vi "PV HLT5xx Valve Test.vi"(6 "Auto/Manual in":bool[](array[boolean]), 7 "Adress of unit":u16=1 min=1 max=999 step=1, 8 "error in (no error)":errorcluster, 9 "On/Off in":bool[](array[boolean]), 10 "Parameter\nread only<->describe":bool, 11 "VISA session":refnum<visa-resource-name>) -> (0 "error out":errorcluster, 1 "On/Off out":bool[](array[boolean]), 2 "response (data)":string, 3 "dup VISA session":refnum<visa-resource-name>, 4 "Auto/Manual out":bool[](array[boolean]))   [LabVIEW 2016, in "Pfeiffer Vacuum.lvlib"]
doc: "This VI allows you to set or check the Valve \"Valve test (Para 609)\" on the SmartTest (HLT5xx)."
uses:
  Pfeiffer Vacuum.lvlib
panel:
  # "Valve test"
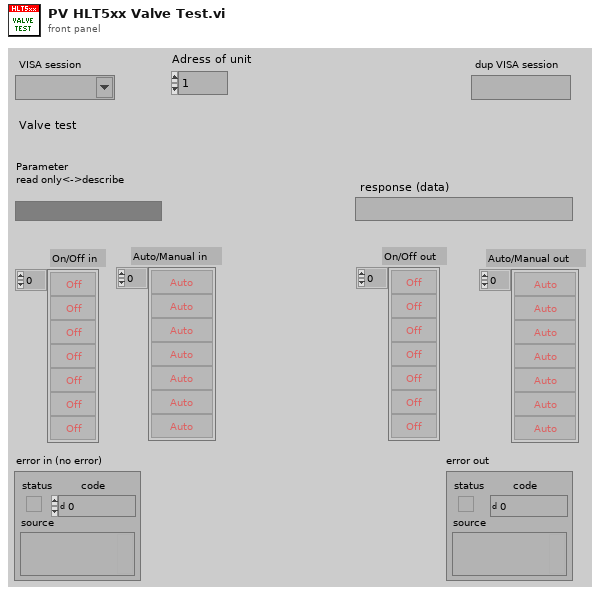
[diagram p1: front panel]
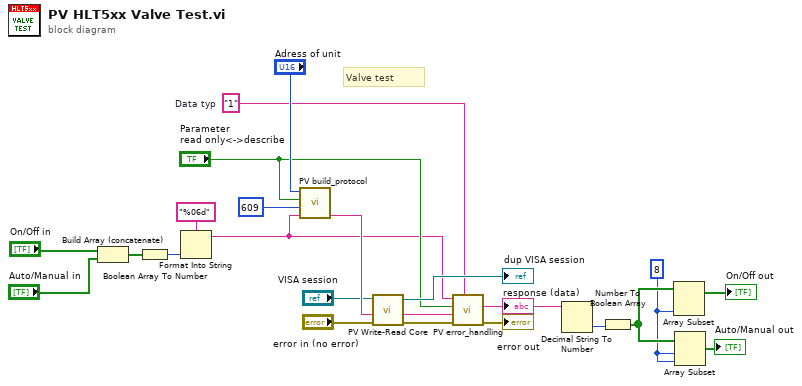
[diagram p0: block diagram]
diagram:
  w17 = "1"  # Data typ
  w10 = 8 ("Länge")
  # "Valve test"
  n1 = Build Array (concatenate)("On/Off in", "Auto/Manual in") -> (w4:bool[])
  n2 = Boolean Array To Number(Boolean array=w4) -> (number=w2:u32)
  n3 = Format Into String(format string="%06d" ("Format-String"), w2) -> (resulting string=w1:string)  [unwired: 2 in, 1 out]
  n4 = call "PV build_protocol.vi"("Data"=w1, "Parameter-number"=u16 609, "parameter\nread<->describe"="Parameter\nread only<->describe", "Adress"="Adress of unit") -> ("output"=w21:string)  [unwired: 3 in]
  n5 = call "PV Write-Read Core.vi"("error in"="error in (no error)", "Write data in"=w21, "VISA session"="VISA session") -> ("error out"=w19:errorcluster, "response (data) out"=w20:string, "dup VISA session"=→"dup VISA session":refnum<visa-resource-name>)  [unwired: 2 in]
  n6 = call "PV error_handling.vi"("Data Typ in"=w17, "error in"=w19, "response (data) in"=w20, "Parameter\nread only<->describe"="Parameter\nread only<->describe", "data in"=w1) -> ("error out"=→"error out":errorcluster, "Data out"=w8:string)  [unwired: 4 in, 1 out]
  "response (data)" <- w8
  n7 = Decimal String To Number(string=w8) -> (number=w12:i32)  [unwired: 2 in, 1 out]
  n8 = Number To Boolean Array(number=w12) -> (Boolean array=w11:bool[])
  n9 = Array Subset(array=w11, length=w10) -> (→"On/Off out":bool[])  [unwired: 1 in]
  n10 = Array Subset(array=w11, index=w10, length=w10) -> (→"Auto/Manual out":bool[])
